vi "ExecuteRole.vi"(0 "object in":refnum<class "PrimaryAttackerRole.lvclass">, 2 "Robot in":refnum<class "Robot.lvclass">, 3 "GameRef":refnum<data-value>, 5 "error in (no error)":errorcluster) -> (14 "object out":refnum<class "PrimaryAttackerRole.lvclass">, 16 "Robot out":refnum<class "Robot.lvclass">, 19 "error out":errorcluster)   [LabVIEW 2023, in "PrimaryAttackerRole.lvclass"]
uses:
  PrimaryAttackerRole.lvclass
  Robot_class/Robot.lvclass
  Game_class/Game.lvclass
  NewSTP/NewRoles/Role_v2_class/Role_v2.lvclass
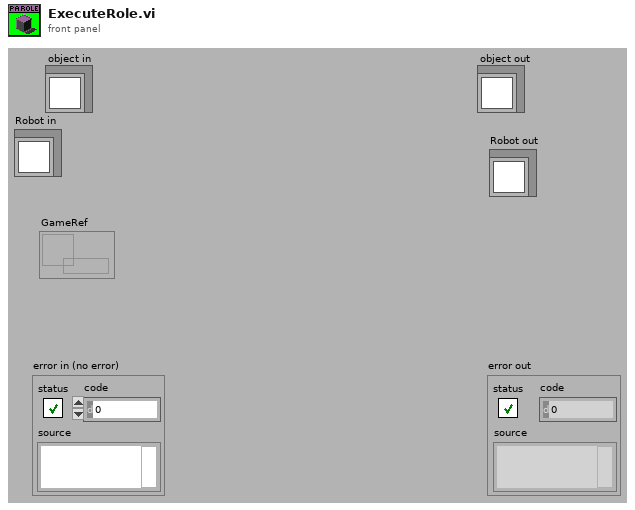
[diagram p1: front panel]
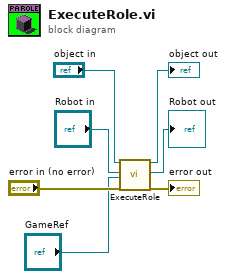
[diagram p0: block diagram]
diagram:
  n1 = call-parent "ExecuteRole.vi"("object in"="object in", "Robot in"="Robot in", "GameRef"="GameRef", "error in (no error)"="error in (no error)") -> ("object out"=→"object out":refnum<class "PrimaryAttackerRole.lvclass">, "Robot out"=→"Robot out":refnum<class "Robot.lvclass">, "error out"=→"error out":errorcluster)  [unwired: 13 in]
